vi "GLOBAL_TDC_Data.vi"(4 "State":enum16{"Initialise", "Write", "Read"}(ring), 5 "Data In":cluster{"Channel":u8, "TDC Data":u16}[](array[cluster])) -> (1 "Valid Read?":bool, 2 "Data Out":cluster{"Channel":u8, "TDC Data":u16}[](array[cluster]))   [LabVIEW 2014]
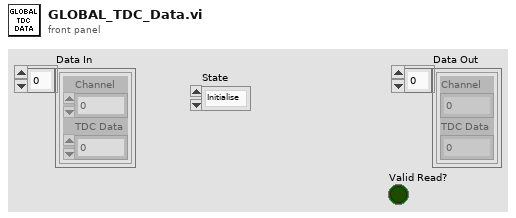
[diagram p1: front panel]
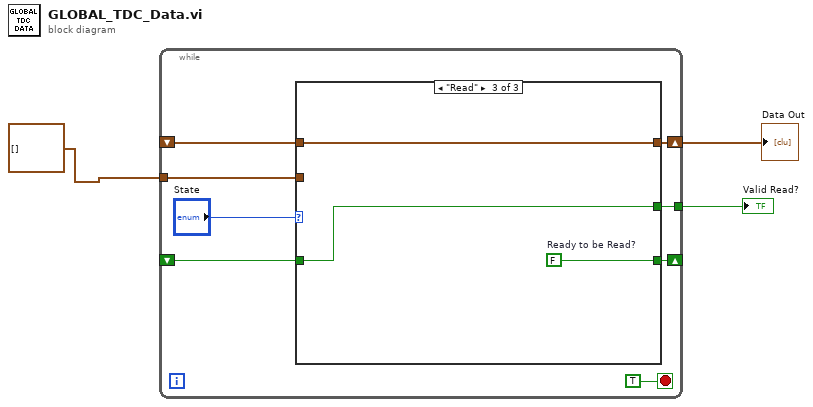
[diagram p0: block diagram]
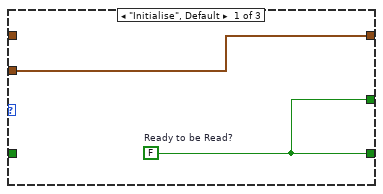
[diagram p2: hidden frame]
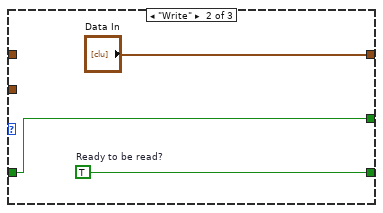
[diagram p3: hidden frame]
diagram:
  n1 = while {
    tunnel: cluster{"Channel":u8, "TDC Data":u16}[] [] -> [w10]
    shift-right: [w9] -> w3
    shift-left: _ -> [w8]
    shift-right: [w6] -> _
    shift-left: _ -> [w5]
    tunnel: [w4] -> w1
    stop <- TRUE stop-if-true
    n2 = case shown="\"Read\"" "State" {
      tunnel: w10 -> [w12 _ _]
      tunnel: [w12 "Data In" w18] -> w9
      tunnel: w8 -> [_ _ w18]
      tunnel: [w13 w15 w19] -> w6
      tunnel: w5 -> [_ w14 w17]
      tunnel: [w13 w14 w17] -> w4
      frame "Initialise", Default {
        w13 = FALSE  # Ready to be Read?
      }
      frame "Write" {
        w15 = TRUE  # Ready to be read?
      }
      frame "Read" {
        w19 = FALSE  # Ready to be Read?
      }
    }
  }
  "Data Out" <- w3
  "Valid Read?" <- w1
